vi "Read Configuration.vi"(8 "error in":errorcluster, 11 "Ballard MIL-STD 1553 custom device in":T1 format="%.0x") -> (0 "error out":errorcluster, 2 "1553 channels":T2[](array[typedef]), 3 "Ballard MIL-STD 1553 custom device out":T1 format="%.0x")   [LabVIEW 2020, in "AIM MIL-STD-1553 Scripting.lvlib"]
uses:
  AIM MIL-STD-1553 Scripting.lvlib
  <vilib>/NI VeriStand/Custom Device API/Custom Device Item Ref.ctl
  Shared/1553 Channel.ctl
  Shared/Address.ctl
  Shared/Message Definition.ctl
  Shared/Message Type.ctl
  Shared/Terminal Endpoint.ctl
  Shared/Parameter Definition.ctl
  <vilib>/NI VeriStand/Custom Device API/Custom Device API.lvlib
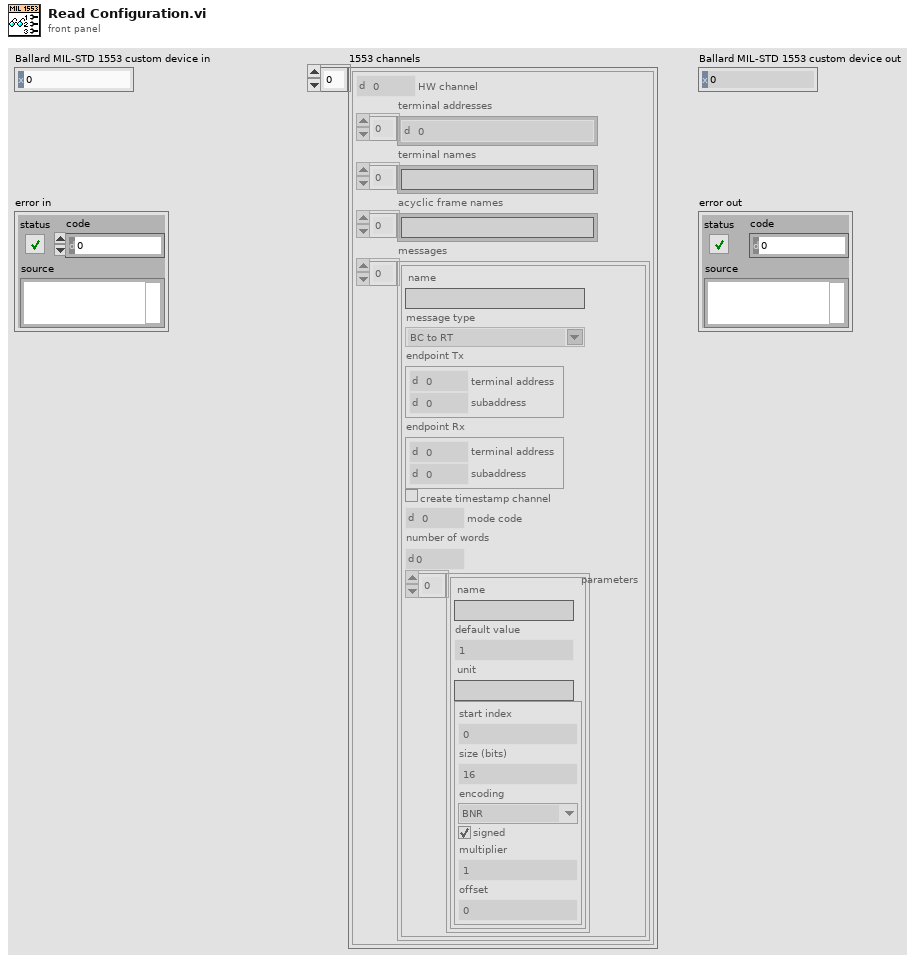
[diagram p1: front panel]
types:
  T1 = typedef "Custom Device API.lvlib/Custom Device Item Ref.ctl" = u64
  T2 = typedef "1553 Channel.ctl" = cluster{"HW channel":u16, "terminal addresses":T3[], "terminal names":string[], "acyclic frame names":string[], "messages":T4[]}
  T3 = typedef "Address.ctl" = u16
  T4 = typedef "Message Definition.ctl" = cluster{"name":string, "message type":T5, "endpoint Tx":T6, "endpoint Rx":T6, "create timestamp channel":bool, "mode code":u16, "number of words":u16, "parameters":cluster{"name":string, "default value":dbl, "unit":string, "parameter definition":T7}[]}
  T5 = typedef "Message Type.ctl" = string
  T6 = typedef "Terminal Endpoint.ctl" = cluster{"terminal address":T3, "subaddress":T3}
  T7 = typedef "Parameter Definition.ctl" = cluster{"start index":i32, "size (bits)":i32, "encoding":enum16{"BNR", "BCD", "Discrete"}, "signed":bool, "multiplier":dbl, "offset":dbl}
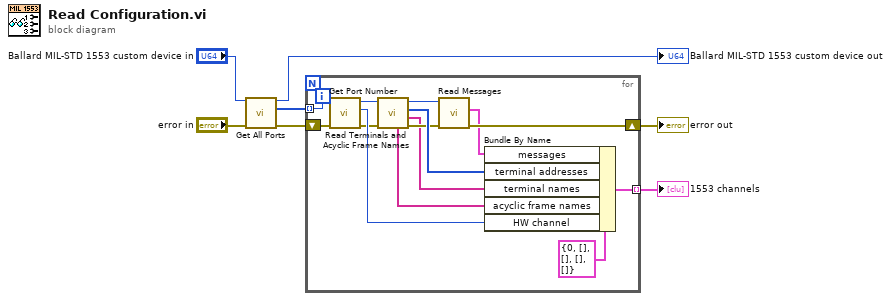
[diagram p0: block diagram]
diagram:
  n1 = call "Get All Ports.vi"("error in"="error in", "Ballard MIL-STD 1553 custom device in"="Ballard MIL-STD 1553 custom device in") -> ("error out"=w4:errorcluster, "ports"=w3:T1[], "Ballard MIL-STD 1553 custom device out"=→"Ballard MIL-STD 1553 custom device out":T1)  [unwired: 7 in]
  n2 = for {
    shift-right: [w10] -> w7
    shift-left: w4 -> [w21]
    tunnel: w3 -> [w20] mode=indexing
    tunnel: [w17] -> w1 mode=indexing
    n3 = call "Get Port Number.vi"("error in"=w21, "port in"=w20) -> ("error out"=w15:errorcluster, "port number"=w18:u16, "port out"=w16:T1)  [unwired: 6 in, 1 out]
    n4 = call "Read Terminals and Acyclic Frame Names.vi"("error in"=w15, "port in"=w16) -> ("error out"=w11:errorcluster, "terminal names"=w8:string[], "terminals"=w14:T3[], "port out"=w12:T1, "acyclic frame names"=w13:string[])  [unwired: 5 in]
    n5 = call "Read Messages.vi"("error in"=w11, "port in"=w12) -> ("error out"=w10:errorcluster, "messages"=w9:T4[])  [unwired: 7 in, 1 out]
    n6 = Bundle By Name(cluster=T2 {"HW channel"=0, "terminal addresses"=[], "terminal names"=[], "acyclic frame names"=[], "messages"=[]} ("1553 channel"), "messages"=w9, "terminal addresses"=w14, "terminal names"=w8, "acyclic frame names"=w13, "HW channel"=w18) -> (w17:T2)
  }
  "error out" <- w7
  "1553 channels" <- w1
